vi "Check if configuration files exist.vi"(8 "error in (no error)":errorcluster, 11 "ThorcamBase in":refnum<class "Thorcam.lvclass">) -> (0 "error out":errorcluster, 2 "configuration file exists?":bool, 3 "ThorcamBase out":refnum<class "Thorcam.lvclass">)   [LabVIEW 2012, in "Thorcam.lvclass"]
doc: "Checks whether all required configuration files for the component exist."
uses:
  Thorcam.lvclass
  <vilib>/Distrio/Murmex/Murmex/Murmex.lvclass
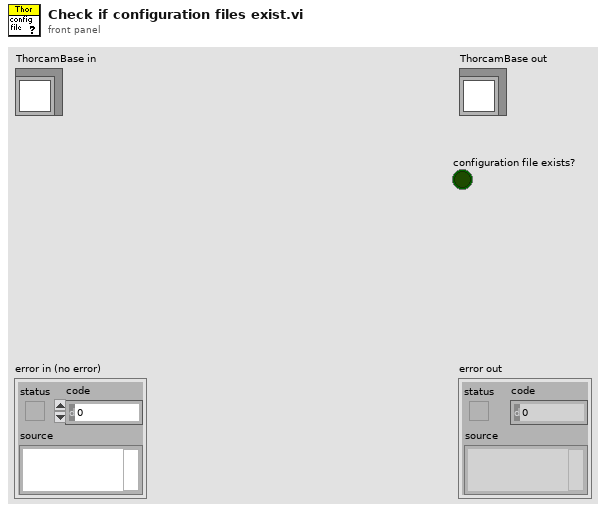
[diagram p1: front panel]
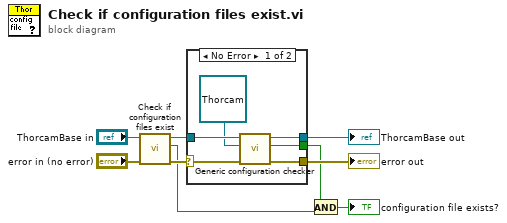
[diagram p0: block diagram]
diagram:
  n1 = call-parent "Check if configuration files exist.vi"("error in (no error)"="error in (no error)", "MurmexBase in"="ThorcamBase in") -> ("error out"=w7:errorcluster, "configuration file exists?"=w3:bool, "MurmexBase out"=w6:refnum<class "Thorcam.lvclass">)  [unwired: 7 in]
  n2 = case shown="No Error" w7 {
    selector: w7 -> [w15 w16]
    tunnel: w6 -> [w13 w17]
    tunnel: [w14 w16] -> w5
    tunnel: [w11 w17] -> w4
    tunnel: [w10 _] -> w1
    frame No Error {
      n3 = call <vilib>:"Generic configuration checker.vi"("error in (no error)"=w15, "inheritance level"=refnum<class "Thorcam.lvclass"> refnum ("Thorcam"), "Murmex in"=w13) -> ("error out"=w14:errorcluster, "configuration file exists?"=w10:bool, "Murmex out"=w11:refnum<class "Thorcam.lvclass">)  [unwired: 6 in]
    }
    frame Error {
    }
  }
  "error out" <- w5
  "ThorcamBase out" <- w4
  n4 = And(x=w1, y=w3) -> (x .and. y?=→"configuration file exists?":bool)
